vi "Websockets_Test Disconnected by Peer.vi"(8 "error in (no error)":errorcluster) -> (0 "error out":errorcluster)   [LabVIEW 2013]
uses:
  <vilib>/addons/_JKI Toolkits/Caraya/classes/Assert/Assert Not Error.vi
  <vilib>/addons/_JKI Toolkits/Caraya/classes/Assert/Assert Equal Value_Variant.vi
  <vilib>/addons/_JKI Toolkits/Caraya/classes/Test/Test.lvclass
  <vilib>/addons/_JKI Toolkits/Caraya/classes/Assert/Assert.lvclass
  <vilib>/LabVIEW Open Source Project/Connection/Connection/Connection.lvclass
  source/MQTT_Websockets/Connection/WebsocketsConnection.lvclass
panel:
  out "connected":bool
  out "server connected":bool
  out "client connected":bool
  out "Comm OK":bool
  out "value":dbl
  out "Bytes":u8[](array[numeric]) format="%08b"
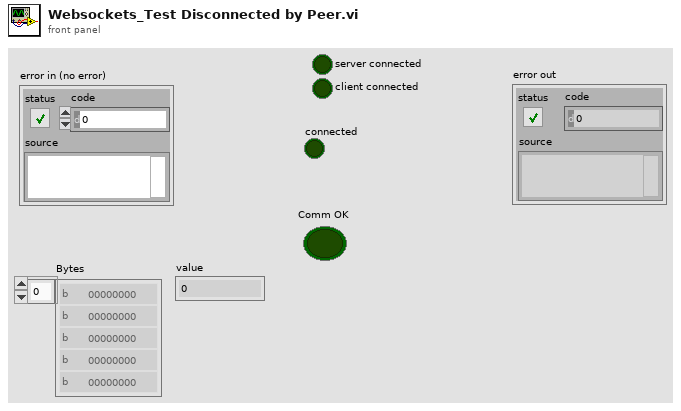
[diagram p1: front panel]
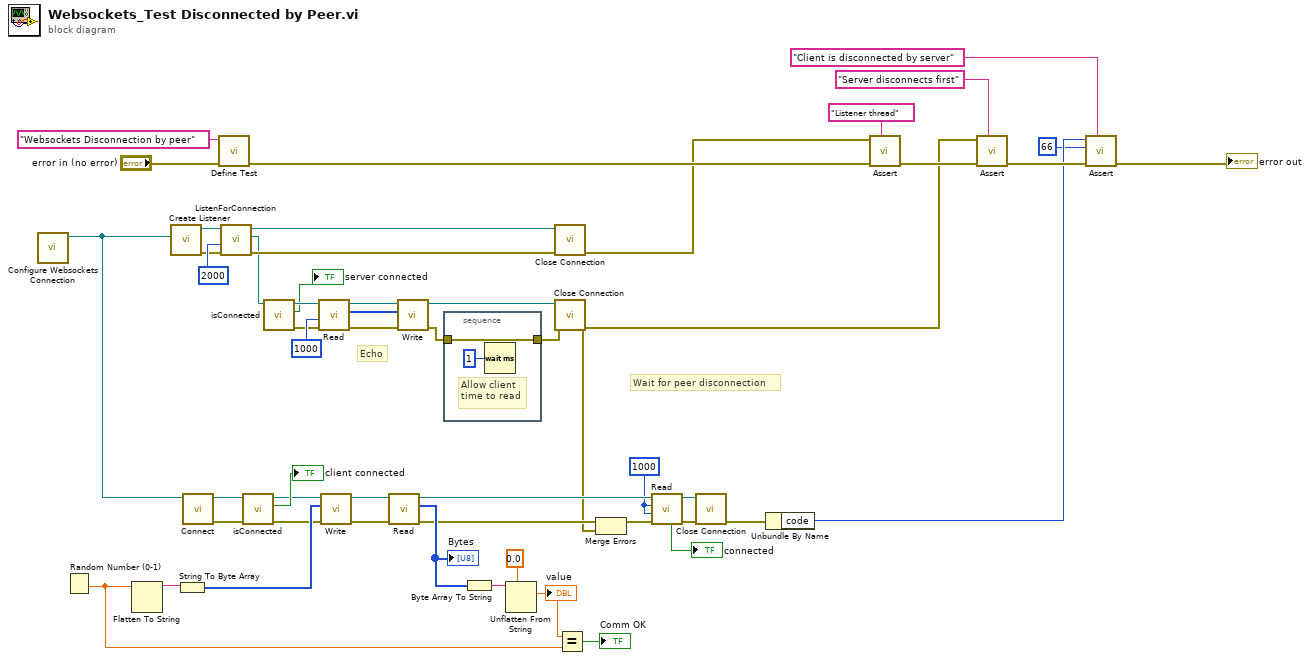
[diagram p0: block diagram]
diagram:
  w11 = 1000 ("bytes to read (100)")
  # "Wait for peer disconnection"
  # "Echo"
  n1 = call "Configure Websockets Connection.vi"() -> ("WSConnection"=w1:refnum<class "WebsocketsConnection.lvclass">)  [unwired: 10 in, 1 out]
  n2 = Random Number (0-1)() -> (number: 0 to 1=w26:dbl)
  n3 = Flatten To String(anything=w26) -> (data string=w33:string)  [unwired: 3 in, 2 out]
  n4 = call <vilib>:"Create Listener.vi"("Connection Configuration"=w1) -> ("error out"=w41:errorcluster, "Listener"=w44:refnum<class "WebsocketsConnection.lvclass">)  [unwired: 9 in]
  n5 = String To Byte Array(string=w33) -> (unsigned byte array=w32:u8[])
  n6 = call <vilib>:"Connect.vi"("Connection in"=w1) -> ("error out"=w21:errorcluster, "Connection out"=w19:refnum<class "WebsocketsConnection.lvclass">)  [unwired: 9 in]
  n7 = call <vilib>:"Define Test.vi"("error in (no error)"="error in (no error)", "Label (VI Title)"="Websockets Disconnection by peer") -> ("error out"=w52:errorcluster)  [unwired: 9 in]
  n8 = call <vilib>:"ListenForConnection.vi"("error in (no error)"=w41, "timeout (2000 ms)"=2000 ("bytes to read (100)"), "Listener"=w44) -> ("error out"=w28:errorcluster, "Connection"=w17:refnum<class "Connection.lvclass">, "Listener out"=w42:refnum<class "WebsocketsConnection.lvclass">)  [unwired: 5 in, 1 out]
  n9 = call <vilib>:"isConnected.vi"("error in (no error)"=w21, "Connection in"=w19) -> ("error out"=w20:errorcluster, "connected"=→"client connected":bool, "Connection out"=w18:refnum<class "WebsocketsConnection.lvclass">)  [unwired: 7 in]
  n10 = call <vilib>:"isConnected.vi"("Connection in"=w17) -> ("error out"=w15:errorcluster, "connected"=→"server connected":bool, "Connection out"=w16:refnum<class "Connection.lvclass">)  [unwired: 8 in]
  n11 = call <vilib>:"Read.vi"("error in (no error)"=w15, "timeout (2000 ms)"=1000 ("bytes to read (100)"), "TCPConnection in"=w16) -> ("error out"=w36:errorcluster, "Bytes"=w38:u8[], "TCPConnection out"=w39:refnum<class "Connection.lvclass">)  [unwired: 4 in, 2 out]
  n12 = call <vilib>:"Write.vi"("error in (no error)"=w20, "Bytes"=w32, "Connection in"=w18) -> ("error out"=w35:errorcluster, "Connection"=w37:refnum<class "WebsocketsConnection.lvclass">)  [unwired: 7 in]
  n13 = call <vilib>:"Read.vi"("error in (no error)"=w35, "TCPConnection in"=w37) -> ("error out"=w7:errorcluster, "Bytes"=w31:u8[], "TCPConnection out"=w13:refnum<class "WebsocketsConnection.lvclass">)  [unwired: 5 in, 2 out]
  "Bytes" <- w31
  n14 = call <vilib>:"Write.vi"("error in (no error)"=w36, "Bytes"=w38, "Connection in"=w39) -> ("error out"=w24:errorcluster, "Connection"=w34:refnum<class "Connection.lvclass">)  [unwired: 7 in]
  n15 = stacked-sequence {
    tunnel: w24 -> [w54]
    tunnel: [w54] -> w23
    frame #0 {
      # "Allow client\ntime to read"
      n16 = Wait (ms)(milliseconds to wait=u32 1) -> ()  [unwired: 1 out]
    }
  }
  n17 = Byte Array To String(unsigned byte array=w31) -> (string=w30:string)
  n18 = Unflatten From String(type=0.0, binary string=w30) -> (value=w27:dbl)  [unwired: 3 in, 2 out]
  "value" <- w27
  n19 = call <vilib>:"Close Connection.vi"("error in (no error)"=w28, "Connection in"=w42) -> ("error out"=w10:errorcluster)  [unwired: 8 in, 1 out]
  n20 = call <vilib>:"Close Connection.vi"("error in (no error)"=w23, "Connection in"=w34) -> ("error out"=w6:errorcluster)  [unwired: 8 in, 1 out]
  n21 = Equal?(x=w27, y=w26) -> (x = y?=→"Comm OK":bool)
  n22 = Merge Errors(w7, w6) -> (w5:errorcluster)
  n23 = call <vilib>:"Read.vi"("error in (no error)"=w5, "timeout (2000 ms)"=w11, "bytes to read (100)"=w11, "TCPConnection in"=w13) -> ("error out"=w8:errorcluster, "TCPConnection out"=w12:refnum<class "WebsocketsConnection.lvclass">, "connected"=→"connected":bool)  [unwired: 3 in, 2 out]
  n24 = call <vilib>:"Close Connection.vi"("error in (no error)"=w8, "Connection in"=w12) -> ("error out"=w9:errorcluster)  [unwired: 8 in, 1 out]
  n25 = Unbundle By Name(w9) -> ("code"=w49:i32)
  n26 = call-poly <vilib>:"Assert.vi"("Label"="Listener thread" ("Label (VI Title)"), "error in (no error)"=w52, "Not Error?"=w10) -> ("error out"=w51:errorcluster)  [unwired: 8 in]
  n27 = call-poly <vilib>:"Assert.vi"("Label"="Server disconnects first" ("Label (VI Title)"), "error in (no error)"=w51, "Not Error?"=w6) -> ("error out"=w50:errorcluster)  [unwired: 8 in]
  n28 = call-poly <vilib>:"Assert.vi"("Label"="Client is disconnected by server" ("Label (VI Title)"), "error in (no error)"=w50, "Y"=66 ("code"), "X"=w49) -> ("error out"=→"error out":errorcluster)  [unwired: 7 in]
